vi "Append Line.vi"(0 "PDF Report IN":refnum<class "PDF Report Class.lvclass">, 1 "Line cluster":T1={"Thickness (point)"=0.75, "Alighment"=enum."Right", "%width"=100.0, "Color"=1, "X Offset (point)"=0.0, "Y Offset (point)"=-6.0} {"%width" min=0 max=100 format="%#.0f"}, 11 "error in (no error)":errorcluster) -> (4 "PDF Report OUT":refnum<class "PDF Report Class.lvclass">, 15 "error out":errorcluster)   [LabVIEW 2019, in "Exaprom PDF.lvlib"]
doc: "<B>ENGLISH</B>\nAppends a <B>horizontal line</B> to the PDF report.\n\n<B>FRANÇAIS</B>\nAjoute une <B>ligne horizontale</B> au rapport PDF.\n\nDeveloped by Jean-Marc Simard\nCopyright © 2010, Exaprom Inc.\nAll rights reserved.\nLicense: BSD\n\nWith iTextSharp 4.1.6 (http://itextsharp.sourceforge.net)\nunder Mozilla Public License Version 1.1\n(http://www.mozilla.org/MPL/MPL-1.1.html)"
uses:
  LV Class/PDF Report Class/PDF Report Class.lvclass
  Controls/General Controls/Line cluster.ctl
  Controls/General Controls/CB SetColor.ctl
  C:/work/niobrara_lv/labview pdf writer fixing/DLL/itextsharp.dll
  DLL/itextsharp.dll
  Exaprom PDF.lvlib
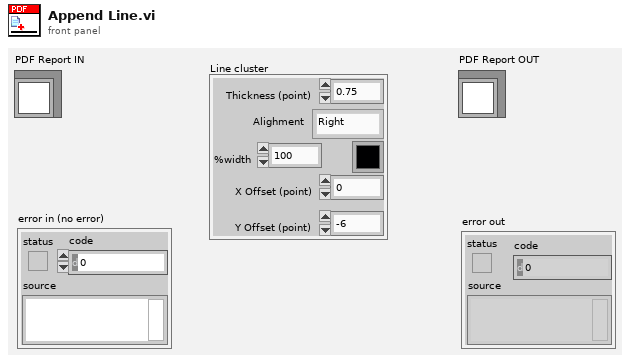
[diagram p1: front panel]
types:
  T1 = typedef "Exaprom PDF.lvlib/Line cluster.ctl" = cluster{"Thickness (point)":sgl, "Alighment":enum16{"Left", "Center", "Right"}, "%width":sgl, "Color":u32, "X Offset (point)":sgl, "Y Offset (point)":sgl}
  T2 = typedef "Exaprom PDF.lvlib/CB SetColor.ctl" = enum16{"Fill", "Stroke"}
  T3 = typedef "Exaprom PDF.lvlib/Page dimensions.ctl" = cluster{"Start at page":i32, "Page Size":T4, "Orientation":T5, "widht":sgl, "height":sgl, "Margin left":sgl, "Margin right":sgl, "Margin top":sgl, "Margin bottom":sgl, "X0":sgl, "X1":sgl, "Y0":sgl, "Y1":sgl}
  T4 = typedef "Exaprom PDF.lvlib/Page size.ctl" = i32
  T5 = typedef "Exaprom PDF.lvlib/Page Orientation.ctl" = enum16{"Portrait", "Landscape"}
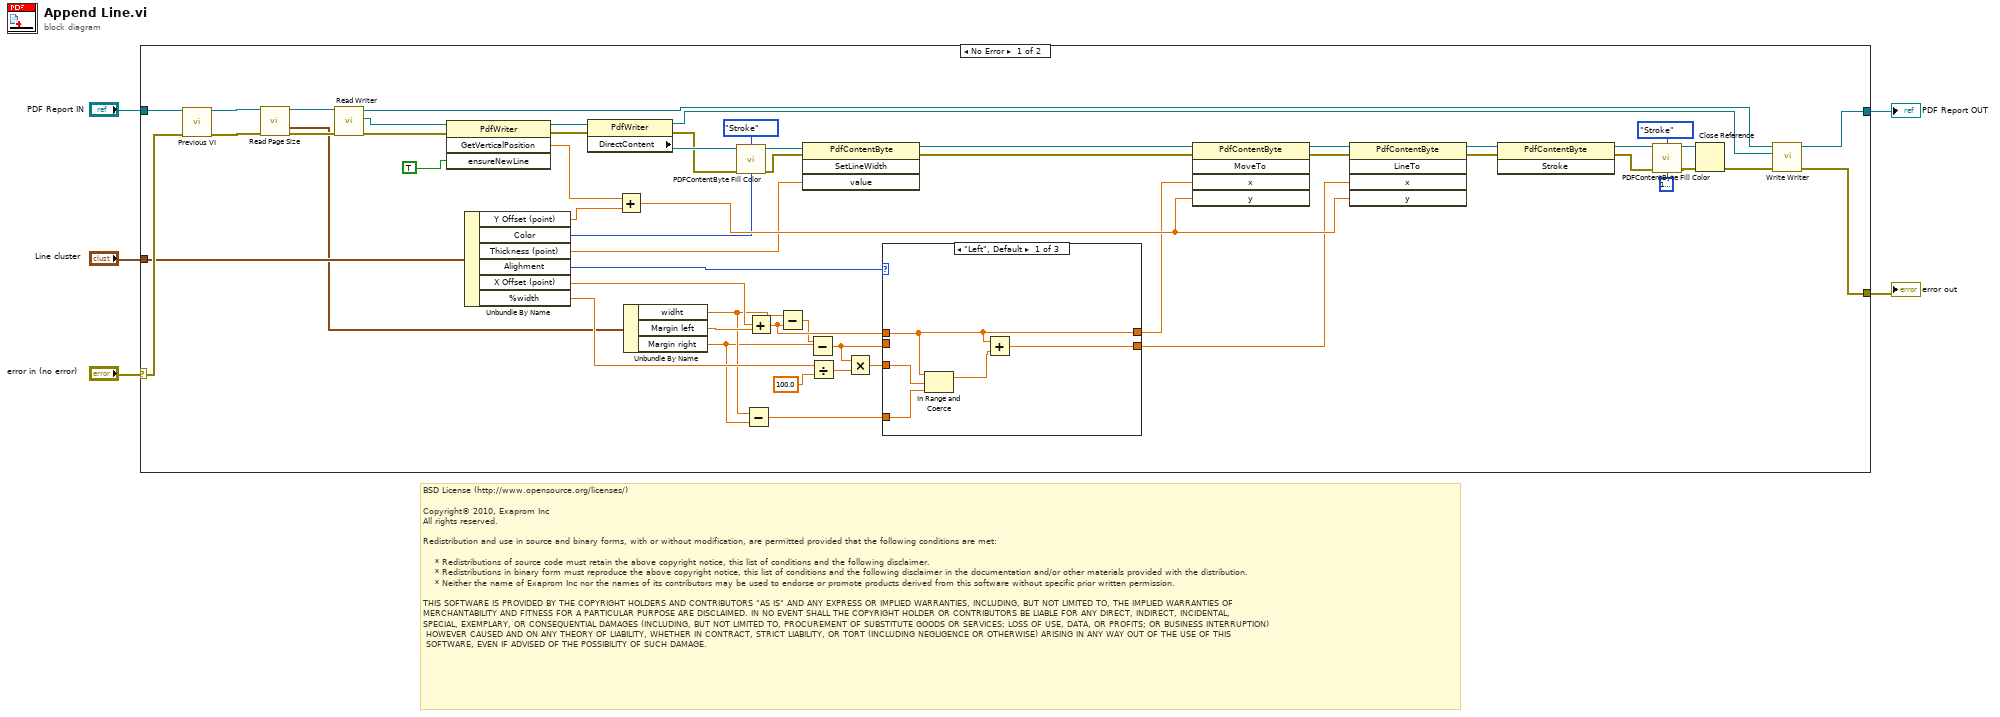
[diagram p0: block diagram]
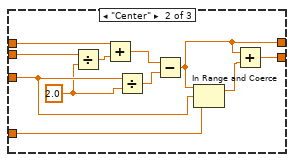
[diagram p2: hidden frame]
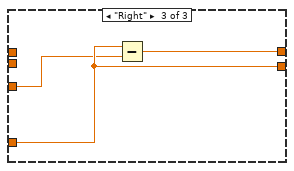
[diagram p3: hidden frame]
diagram:
  # "BSD License (http://www.opensource.org/licenses/)\n\nCopyright© 2010, Exaprom Inc\nAll rights reserved.\n\nRedistribution and use in source and binary forms, with or without modification, are permitted provided that the following conditions are met:\n\n    * Redistributions of source code must retain the above copyright notice, this list of conditions and the following disclaimer.\n    * Redistributions in binary form must reproduce the above copyright notice, this list of conditions and the following disclaimer in the documentation and/or other materials provided with the distribution.\n    * Neither the name of Exaprom Inc nor the names of its contributors may be used to endorse or promote products derived from this software without specific prior written permission.\n\nTHIS SOFTWARE IS PROVIDED BY THE COPYRIGHT HOLDERS AND CONTRIBUTORS \"AS IS\" AND ANY EXPRESS OR IMPLIED WARRANTIES, INCLUDING, BUT NOT LIMITED TO, THE IMPLIED WARRANTIES OF \nMERCHANTABILITY AND FITNESS FOR A PARTICULAR PURPOSE ARE DISCLAIMED. IN NO EVENT SHALL THE COPYRIGHT HOLDER OR CONTRIBUTORS BE LIABLE FOR ANY DIRECT, INDIRECT, INCIDENTAL,\nSPECIAL, EXEMPLARY, OR CONSEQUENTIAL DAMAGES (INCLUDING, BUT NOT LIMITED TO, PROCUREMENT OF SUBSTITUTE GOODS OR SERVICES; LOSS OF USE, DATA, OR PROFITS; OR BUSINESS INTERRUPTION)\n HOWEVER CAUSED AND ON ANY THEORY OF LIABILITY, WHETHER IN CONTRACT, STRICT LIABILITY, OR TORT (INCLUDING NEGLIGENCE OR OTHERWISE) ARISING IN ANY WAY OUT OF THE USE OF THIS\n SOFTWARE, EVEN IF ADVISED OF THE POSSIBILITY OF SUCH DAMAGE."
  n1 = case shown="No Error" "error in (no error)" {
    selector: "error in (no error)" -> [w60 w81]
    tunnel: [w9 w81] -> w5
    tunnel: "PDF Report IN" -> [w30 w80]
    tunnel: [w7 w80] -> w2
    tunnel: "Line cluster" -> [w45 _]
    frame No Error {
      n2 = call "Previous VI.vi"("PDF Report IN"=w30, "error in (no error)"=w60) -> ("PDF Report OUT"=w14:refnum<class "PDF Report Class.lvclass">, "error out"=w13:errorcluster)  [unwired: 12 out]
      n3 = call "Read Page Size.vi"("PDF Report"=w14, "error in (no error)"=w13) -> ("PDF Report duplicate"=w11:refnum<class "PDF Report Class.lvclass">, "Page (points)"=w28:T3, "error out"=w29:errorcluster)  [unwired: 11 out]
      n4 = call-dynamic "Read Writer.vi"("error in (no error)"=w29, "PDF Report Class in"=w11) -> ("error out"=w12:errorcluster, "Writer"=w10:refnum<k24>, "PDF Report Class out"=w6:refnum<class "PDF Report Class.lvclass">)  [unwired: 7 in]
      n5 = invoke class="PdfWriter" method="GetVerticalPosition"(reference=w10, error in=w12, "ensureNewLine"=TRUE) -> (reference out=w58:refnum<k24>, error out=w59:errorcluster, "GetVerticalPosition"=w52:sgl)  [unwired: 1 in, 1 out]
      n6 = Unbundle By Name(w45) -> ("Y Offset (point)"=w44:sgl, "Color"=w17:u32, "Thickness (point)"=w43:sgl, "Alighment"=w41:enum16{"Left", "Center", "Right"}, "X Offset (point)"=w39:sgl, "%width"=w42:sgl)
      n7 = property class="PdfWriter"(reference=w58, error in=w59) -> (reference out=w8:refnum<k24>, error out=w19:errorcluster, "DirectContent"=w20:refnum<k24>)
      n8 = Add(x=w52, y=w44) -> (x+y=w51:sgl)
      n9 = Unbundle By Name(w28) -> ("widht"=w37:sgl, "Margin left"=w40:sgl, "Margin right"=w35:sgl)
      n10 = call "PDFContentByte Fill Color.vi"("PDFContentByte"=w20, "CB SetColor"=CB_SetColor."Stroke", "error in (no error)"=w19, "Color Box"=w17) -> ("PDFContentByte duplicate"=w21:refnum<k24>, "error out"=w18:errorcluster)  [unwired: 10 out]
      n11 = Subtract(x=w37, y=w35) -> (x-y=w36:sgl)
      n12 = Add(x=w39, y=w40) -> (x+y=w38:sgl)
      n13 = Subtract(x=w37, y=w38) -> (x-y=w34:sgl)
      n14 = invoke class="PdfContentByte" method="SetLineWidth"(reference=w21, error in=w18, "value"=w43) -> (reference out=w32:refnum<k24>, error out=w31:errorcluster)  [unwired: 1 in, 2 out]
      n15 = Subtract(x=w34, y=w35) -> (x-y=w33:sgl)
      n16 = Divide(x=w42, y=sgl 100.0) -> (x/y=w46:sgl)
      n17 = Multiply(x=w33, y=w46) -> (x*y=w49:sgl)
      n18 = case shown="\"Left\", Default" w41 {
        tunnel: w38 -> [w63 w72 _]
        tunnel: [w63 w69 w78] -> w50
        tunnel: w49 -> [w62 w68 w77]
        tunnel: [w65 w76 w79] -> w48
        tunnel: w36 -> [w64 w67 w79]
        tunnel: w33 -> [_ w74 _]
        frame "Left", Default {
          n19 = In Range and Coerce(upper limit=w63, x=w62, lower limit=w64) -> (coerced(x)=w61:sgl)  [unwired: 1 out]
          n20 = Add(x=w63, y=w61) -> (x+y=w65:sgl)
        }
        frame "Center" {
          w66 = sgl 2.0 ("y")
          n21 = Divide(x=w74, y=w66) -> (x/y=w73:sgl)
          n22 = Add(x=w72, y=w73) -> (x+y=w70:sgl)
          n23 = Divide(x=w68, y=w66) -> (x/y=w71:sgl)
          n24 = Subtract(x=w70, y=w71) -> (x-y=w69:sgl)
          n25 = In Range and Coerce(upper limit=w69, x=w68, lower limit=w67) -> (coerced(x)=w75:sgl)  [unwired: 1 out]
          n26 = Add(x=w69, y=w75) -> (x+y=w76:sgl)
        }
        frame "Right" {
          n27 = Subtract(x=w79, y=w77) -> (x-y=w78:sgl)
        }
      }
      n28 = invoke class="PdfContentByte" method="MoveTo"(reference=w32, error in=w31, "x"=w50, "y"=w51) -> (reference out=w53:refnum<k24>, error out=w56:errorcluster)  [unwired: 1 in, 3 out]
      n29 = invoke class="PdfContentByte" method="LineTo"(reference=w53, error in=w56, "x"=w48, "y"=w51) -> (reference out=w54:refnum<k24>, error out=w55:errorcluster)  [unwired: 1 in, 3 out]
      n30 = invoke class="PdfContentByte" method="Stroke"(reference=w54, error in=w55) -> (reference out=w25:refnum<k24>, error out=w26:errorcluster)  [unwired: 1 in, 1 out]
      n31 = call "PDFContentByte Fill Color.vi"("PDFContentByte"=w25, "CB SetColor"=CB_SetColor."Stroke", "error in (no error)"=w26, "Color Box"=u32 16777222) -> ("PDFContentByte duplicate"=w24:refnum<k24>, "error out"=w23:errorcluster)  [unwired: 10 out]
      n32 = Close Reference(reference=w24, error in (no error)=w23) -> (error out=w27:errorcluster)
      n33 = call-dynamic "Write Writer.vi"("error in (no error)"=w27, "Writer"=w8, "PDF Report Class in"=w6) -> ("error out"=w9:errorcluster, "PDF Report Class out"=w7:refnum<class "PDF Report Class.lvclass">)  [unwired: 7 in]
    }
    frame Error {
    }
  }
  "error out" <- w5
  "PDF Report OUT" <- w2
